vi "GE5565 Write (U64) Cluster.vi"(6 "timeout (1000 ms)":u32=1000, 8 "error in (no error)":errorcluster, 9 "buffer":dbl[](array[numeric]), 10 "offset (0)":u32, 11 "VMIC reference in":T1) -> (0 "error out":errorcluster, 3 "VMIC reference out":T1)   [LabVIEW 2020, in "RefMem DMA Engine.lvlib"]
uses:
  RefMem DMA Engine.lvlib
  <vilib>/Instr/_visa.llb/Select Event Type.ctl
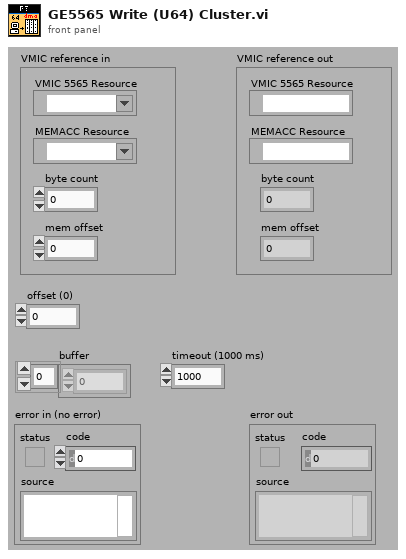
[diagram p1: front panel]
types:
  T1 = cluster{"VMIC 5565 Resource":refnum<visa-resource-name>, "MEMACC Resource":refnum<visa-resource-name>, "byte count":u32, "mem offset":u32}
  T2 = enum16{"big-endian, network order", "native, host order", "little-endian"}
  T3 = typedef "Select Event Type.ctl" = u32
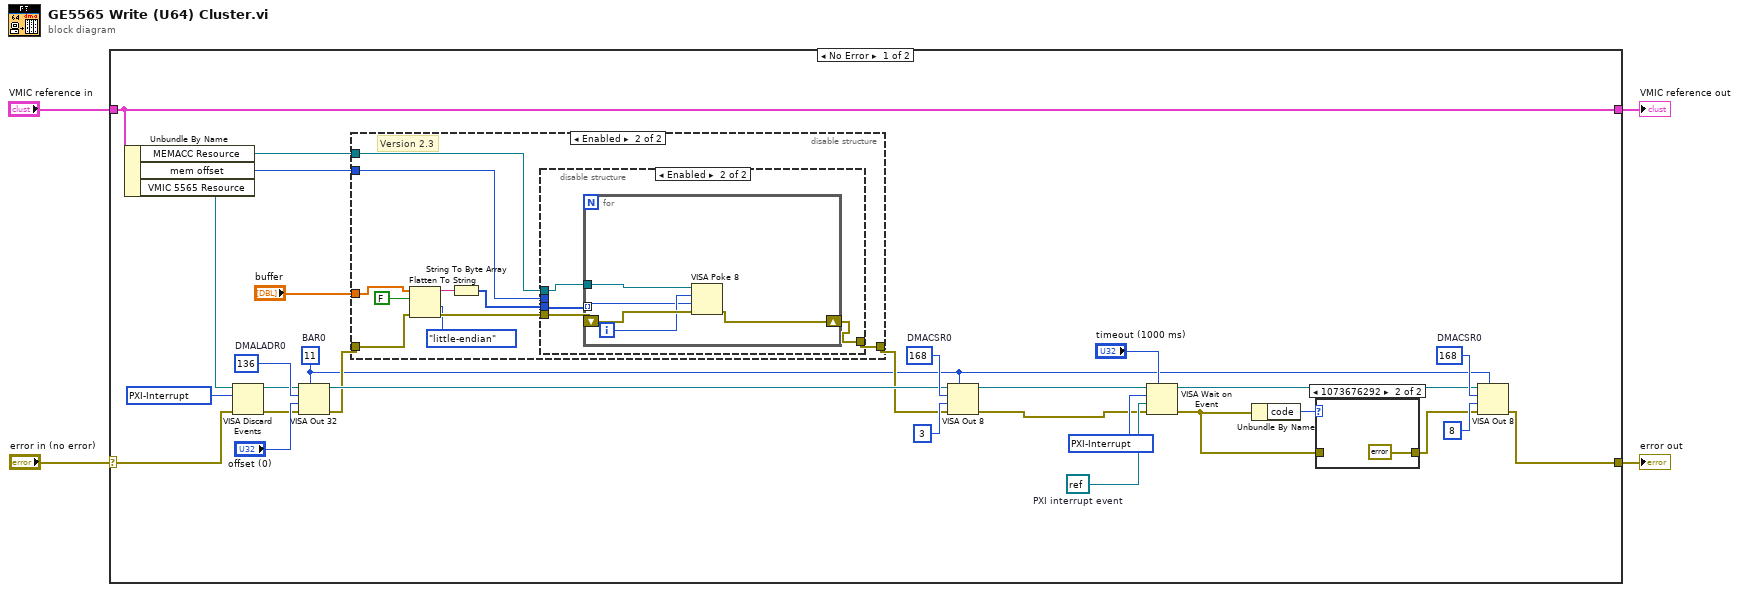
[diagram p0: block diagram]
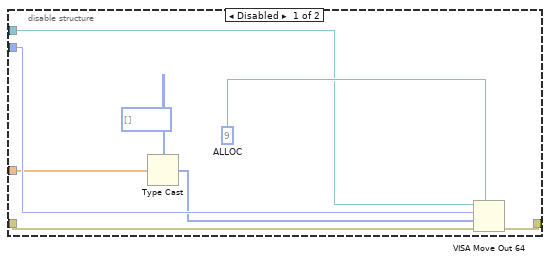
[diagram p2: hidden frame]
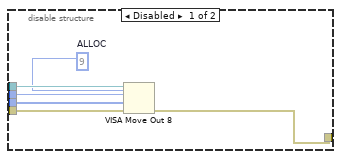
[diagram p3: hidden frame]
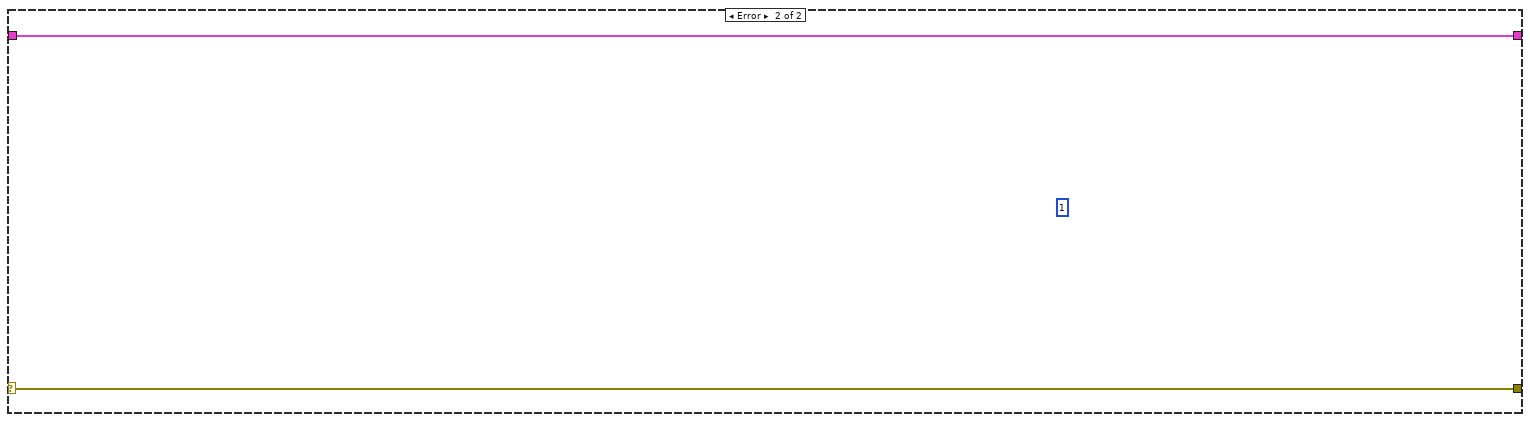
[diagram p5: hidden frame]
diagram:
  n1 = case shown="No Error" "error in (no error)" {
    selector: "error in (no error)" -> [w24 w69]
    tunnel: "VMIC reference in" -> [w15 w70]
    tunnel: [w15 w70] -> w1
    tunnel: [w6 w69] -> w3
    frame No Error {
      w12 = u16 11  # BAR0
      w26 = refnum<visa-resource-name> refnum  # PXI interrupt event
      w14 = u32 168  # DMACSR0
      w21 = T3 1073684514 items=["ServiceRequest"=1073684491, "Trigger"=3221168138, "Clear"=1073684493, "VXI-Signal"=1073684512, "VXI/VME-Interrupt"=3221168161, "VXI/VME-Sysfail"=1073684509, "VXI/VME-Sysreset"=1073684510, "GPIB-CIC"=1073684498, "GPIB-Talk"=1073684499, "GPIB-Listen"=1073684500, "PXI-Interrupt"=1073684514, "AllEnabled"=1073709055] ("Event Type")
      w27 = T3 1073684514 items=["ServiceRequest"=1073684491, "Trigger"=3221168138, "Clear"=1073684493, "VXI-Signal"=1073684512, "VXI/VME-Interrupt"=3221168161, "VXI/VME-Sysfail"=1073684509, "VXI/VME-Sysreset"=1073684510, "GPIB-CIC"=1073684498, "GPIB-Talk"=1073684499, "GPIB-Listen"=1073684500, "PXI-Interrupt"=1073684514, "AllEnabled"=1073709055] ("Event Type")
      w32 = u32 168  # DMACSR0
      w33 = u32 136  # DMALADR0
      n2 = Unbundle By Name(w15) -> ("MEMACC Resource"=w16:refnum<visa-resource-name>, "mem offset"=w17:u32, "VMIC 5565 Resource"=w19:refnum<visa-resource-name>)
      n3 = VISA Discard Events(8:w24, 10:w21, 11:w19) -> (0:w22:errorcluster, 3:w23:refnum<visa-resource-name>)  [unwired: 1 in]
      n4 = VISA Out 32(7:w12, 8:w22, 9:"offset (0)", 10:w33, 11:w23) -> (0:w18:errorcluster, 3:w30:refnum<visa-resource-name>)
      n5 = disable-structure shown="Enabled" {
        disable-tunnel: [w40 w44] -> w20
        disable-tunnel: w18 -> [w39 w46]
        disable-tunnel: w17 -> [w38 w47]
        disable-tunnel: w16 -> [w37 w48]
        disable-tunnel: "buffer" -> [w36 w49]
        frame Disabled {
          w41 = u16 9  # ALLOC
          n6 = Type Cast(type=u64[] [] ("data"), x=w36) -> (*(type *) &x=w34:u64[])
          n7 = VISA Move Out 64(7:w41, 8:w39, 9:w34, 10:w38, 11:w37) -> (0:w40:errorcluster)  [unwired: 1 out]
        }
        frame Enabled {
          # "Version 2.3"
          n8 = Flatten To String(anything=w49, prepend array or string size? (T)=FALSE, byte order (0:big-endian, network order)=T2."little-endian", error in (no error)=w46) -> (data string=w51:string, error out=w45:errorcluster)  [unwired: 1 out]
          n9 = String To Byte Array(string=w51) -> (unsigned byte array=w42:u8[])
          n10 = disable-structure shown="Enabled" {
            disable-tunnel: w42 -> [w57 w60]
            disable-tunnel: w48 -> [w56 w58]
            disable-tunnel: w47 -> [w55 _]
            disable-tunnel: w45 -> [w54 w61]
            disable-tunnel: [w53 w59] -> w44
            frame Disabled {
              w52 = u16 9  # ALLOC
              n11 = VISA Move Out 8(7:w52, 8:w54, 9:w57, 10:w55, 11:w56) -> (0:w53:errorcluster)  [unwired: 1 out]
            }
            frame Enabled {
              n12 = for {
                shift-right: [w65] -> w59
                shift-left: w61 -> [w66]
                tunnel: w60 -> [w62] mode=indexing
                tunnel: w58 -> [w64]
                i -> [w63]
                n13 = VISA Poke 8(8:w66, 9:w62, 10:w63, 11:w64) -> (0:w65:errorcluster)  [unwired: 1 out]
              }
            }
          }
        }
      }
      n14 = VISA Out 8(7:w12, 8:w20, 9:u8 3 ("value (0)"), 10:w32, 11:w30) -> (0:w7:errorcluster, 3:w25:refnum<visa-resource-name>)
      n15 = VISA Wait on Event(7:"timeout (1000 ms)", 8:w7, 9:w26, 10:w27, 11:w25) -> (0:w5:errorcluster, 3:w10:refnum<visa-resource-name>)  [unwired: 2 out]
      n16 = Unbundle By Name(w5) -> ("code"=w8:i32)
      n17 = case shown="1073676292" w8 {
        tunnel: [w67 errorcluster {"status"=FALSE, "code"=0, "source"=""} ("error out")] -> w9
        tunnel: w5 -> [w67 _]
        frame 0, Default {
        }
        frame 1073676292 {
        }
      }
      n18 = VISA Out 8(7:w12, 8:w9, 9:u8 8 ("value (0)"), 10:w14, 11:w10) -> (0:w6:errorcluster)  [unwired: 1 out]
    }
    frame Error {
      (unwired) u32 1
    }
  }
  "error out" <- w3
  "VMIC reference out" <- w1
